vi "MT Generate FSK System Parameters.vi"   [LabVIEW 2020, in "niDMT.lvlib"]
doc: "This VI calculates parameters for use with either the MT Modulate FSK VI or the MT Demodulate FSK VI. The FSK system parameters cluster output from this VI wires to the corresponding input of the FSK modulation or demodulation VI. \n\nThis VI has two polymorphic instances that input either an M-ary value that specifies the number of distinct frequency deviations to use as symbols, or an array of symbol values that explicitly specifies the positions of the symbol map."
uses:
  <vilib>/addons/Modulation/niDMT.lvlib
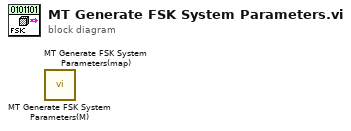
[diagram p0: block diagram]
diagram:
  n1 = call <vilib>:"MT Generate FSK System Parameters(M).vi"() -> ()  [unwired: 13 in, 3 out]
  n2 = call <vilib>:"MT Generate FSK System Parameters(map).vi"() -> ()  [unwired: 13 in, 3 out]
